vi "SubVI_RampingFW+BW_Teleop.vi"(9 "+Speed/s":dbl=0.1 format="%#_13g", 10 "Y Axis Input(Changing Value)":dbl) -> (2 "Y Axis Output":dbl)   [LabVIEW 2017]
panel:
  in  "Number Of Iterations":i32=7
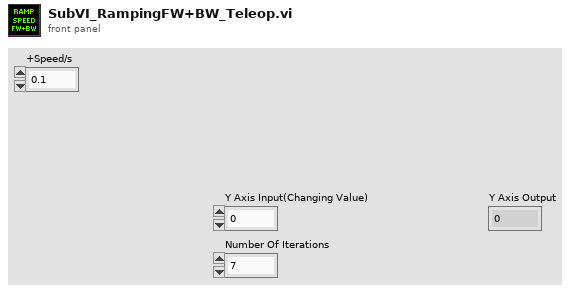
[diagram p1: front panel]
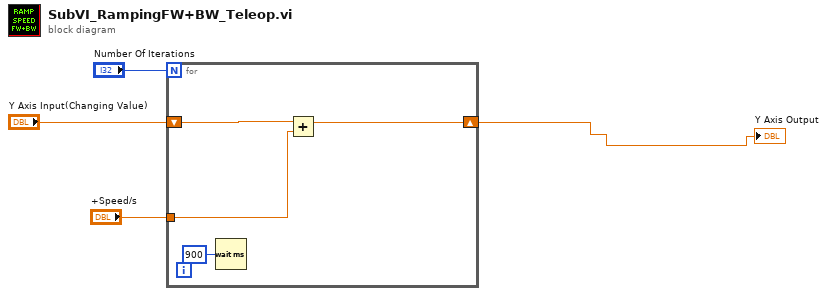
[diagram p0: block diagram]
diagram:
  n1 = for {
    N: "Number Of Iterations" -> [_]
    shift-right: [w6] -> w3
    shift-left: "Y Axis Input(Changing Value)" -> [w8]
    tunnel: "+Speed/s" -> [w5]
    n2 = Wait (ms)(milliseconds to wait=u32 900) -> ()  [unwired: 1 out]
    n3 = Add(x=w8, y=w5) -> (x+y=w6:dbl)
  }
  "Y Axis Output" <- w3
